vi "Dqmh Module.vi"(7 "Config":refnum<class "TAF Proj Config.lvclass">, 8 "error in (no error)":errorcluster, 11 "Library Ref":refnum<vi>) -> (0 "error out":errorcluster, 3 "Dqmh Module out":refnum<class "Dqmh Module.lvclass">)   [LabVIEW 2021, in "TAF Proj Document Type.lvlib" / "Project Parser.lvlib"]
uses:
  <vilib>/Wovalab/AntiDoc/Document Type/Add-ons/LabVIEW TAF Project/Project Parser/Project Parser.lvlib
  <vilib>/Wovalab/AntiDoc/Document Type/Add-ons/LabVIEW TAF Project/Dqmh Module/Dqmh Module.lvclass
  C:/Program Files (x86)/National Instruments/LabVIEW 2021/vi.lib/Wovalab/AntiDoc/Document Type/Add-ons/LabVIEW TAF Project/Lib/Lib.lvclass
  <vilib>/Wovalab/AntiDoc/Document Type/Add-ons/LabVIEW TAF Project/TAF Proj Config/TAF Proj Config.lvclass
  <vilib>/Wovalab/AntiDoc/Document Type/Add-ons/LabVIEW TAF Project/TAF Proj Config/TAF Proj Config.lvclass/TAF Proj Config.ctl
  <vilib>/Wovalab/AntiDoc/Document Type/Add-ons/LabVIEW TAF Project/Dqmh Module/Dqmh Module.lvclass/Dqmh Module.ctl
  <vilib>/Wovalab/AntiDoc/Document Type/Add-ons/LabVIEW TAF Project/TAF Proj Config/Read List Dqmh Default Events.vi
  <vilib>/Wovalab/AntiDoc/Document Type/Add-ons/LabVIEW TAF Project/Dqmh Module/Write Dqmh Module Type.vi
  <vilib>/Wovalab/AntiDoc/Document Type/Add-ons/LabVIEW TAF Project/Dqmh Module/Write Request Link.vi
  <vilib>/Wovalab/AntiDoc/Document Type/Add-ons/LabVIEW TAF Project/Dqmh Module/Write Broadcast Link.vi
  <vilib>/Wovalab/AntiDoc/Document Type/Add-ons/LabVIEW TAF Project/Dqmh Module/Write Request With Reply Links.vi
  <vilib>/Wovalab/AntiDoc/Document Type/Add-ons/LabVIEW TAF Project/Dqmh Module/Write Start Module Callers.vi
  <vilib>/Wovalab/AntiDoc/Document Type/Add-ons/LabVIEW TAF Project/Dqmh Module/Write Stop Module Callers.vi
  <vilib>/Wovalab/AntiDoc/Document Type/Add-ons/LabVIEW TAF Project/Dqmh Module/Write Registred Broadcast.vi
  <vilib>/Wovalab/AntiDoc/Document Type/Add-ons/LabVIEW TAF Project/Dqmh Module/Write Custom Errors.vi
  <vilib>/Wovalab/AntiDoc/Document Type/Add-ons/LabVIEW TAF Project/Dqmh Module/Write Used Requests.vi
  <vilib>/Wovalab/AntiDoc/Document Type/Add-ons/LabVIEW TAF Project/Dqmh Module/Write Used Requests With Reply.vi
  <vilib>/Wovalab/AntiDoc/Document Type/Add-ons/LabVIEW TAF Project/Dqmh Module/Write List Default Event.vi
  <vilib>/Wovalab/AntiDoc/Document Type/Add-ons/LabVIEW TAF Project/Dqmh Event/Dqmh Event.lvclass
  C:/Program Files (x86)/National Instruments/LabVIEW 2021/vi.lib/Wovalab/AntiDoc/Document Type/Add-ons/LabVIEW TAF Project/Vi/Vi.lvclass
  <vilib>/Wovalab/AntiDoc/Document Type/Add-ons/LabVIEW TAF Project/Lib/Lib.lvclass
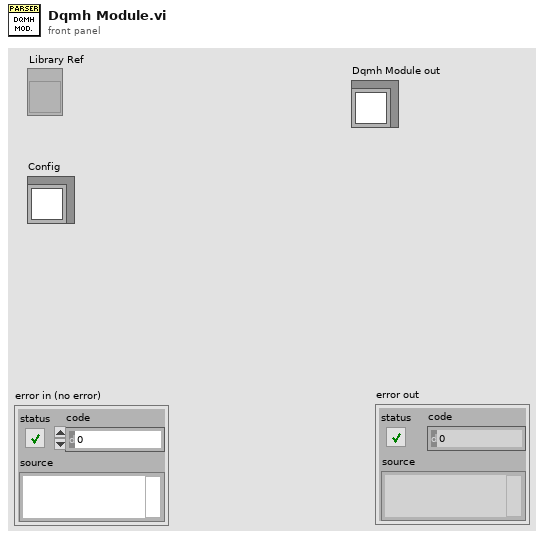
[diagram p1: front panel]
types:
  T1 = typedef "TAF Proj Document Type.lvlib/Project Parser.lvlib/Dqmh Module Info--cluster.ctl" = cluster{"Name":string, "Description":string, "Path":path, "Dqmh Module Type":T2, "Event Info":T3[], "Start Module Info":T3, "Stop Module Info":T3, "Registred Broadcast":T7[], "Custom Errors":T8[], "Used Requests":T9[], "Used Requests With Reply":T9[]}
  T2 = typedef "TAF Proj Document Type.lvlib/Project Parser.lvlib/Dqmh Module Type--enum.ctl" = enum16{"Singleton", "Cloneable"}
  T3 = typedef "TAF Proj Document Type.lvlib/Project Parser.lvlib/Dqmh Event Info--cluster.ctl" = cluster{"Vi Path":path, "Name":string, "Description":string, "Event Type":T4, "Callers":T5[], "Conpane Image":T6}
  T4 = typedef "TAF Proj Document Type.lvlib/Project Parser.lvlib/Dqmh Event Type--enum.ctl" = enum16{"Not a DQMH Event", "Request", "Request And Wait For Reply", "Broadcast"}
  T5 = typedef "TAF Proj Document Type.lvlib/Project Parser.lvlib/Dqmh Event Links--cluster.ctl" = cluster{"Owning Library":string, "Caller":string}
  T6 = typedef "imagedata.ctl" = cluster{"image type":i32, "image depth":i32, "image":u8[], "mask":u8[], "colors":u32[], "Rectangle":cluster{"left":i16, "top":i16, "right":i16, "bottom":i16}}
  T7 = typedef "TAF Proj Document Type.lvlib/Project Parser.lvlib/Module Fonctions--cluster.ctl" = cluster{"Module Name":string, "Functions":string[]}
  T8 = typedef "TAF Proj Document Type.lvlib/Project Parser.lvlib/Custom Error Info.ctl" = cluster{"Code":i32, "Name":string, "Description":string, "Owned by":string}
  T9 = typedef "TAF Proj Document Type.lvlib/Dqmh Module.lvclass/Requests Used By Module--cluster.ctl" = cluster{"Module Name":string, "Request Names":string[]}
  T10 = typedef "TAF Proj Document Type.lvlib/Project Parser.lvlib/Dqmh Event Callers--cluster.ctl" = cluster{"Event Name":string, "Caller Names":string[]}
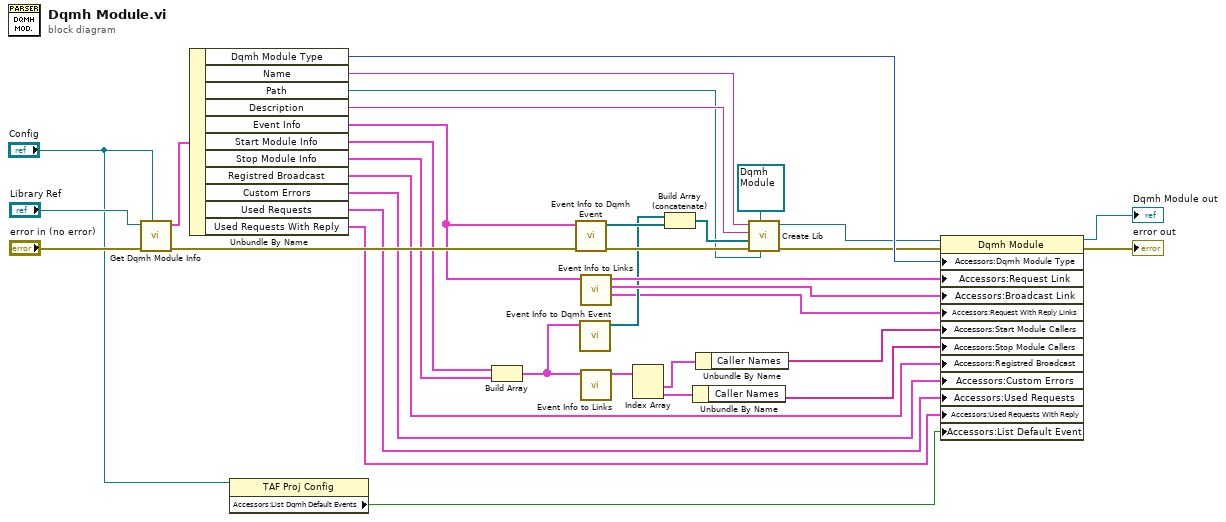
[diagram p0: block diagram]
diagram:
  n1 = call <vilib>:"Get Dqmh Module Info.vi"("Config"="Config", "error in"="error in (no error)", "Library Ref"="Library Ref") -> ("error out"=w28:errorcluster, "Dqmh Module Info"=w35:T1)  [unwired: 7 in]
  n2 = Unbundle By Name(w35) -> ("Dqmh Module Type"=w29:T2, "Name"=w33:string, "Path"=w8:path, "Description"=w32:string, "Event Info"=w26:T3[], "Start Module Info"=w21:T3, "Stop Module Info"=w20:T3, "Registred Broadcast"=w9:T7[], "Custom Errors"=w7:T8[], "Used Requests"=w2:T9[], "Used Requests With Reply"=w1:T9[])
  n3 = property class="TAF Proj Config"(reference="Config") -> ("Accessors:List Dqmh Default Events"=w3:bool)  [unwired: 1 in, 2 out]
  n4 = Build Array(w21, w20) -> (w14:T3[])
  n5 = call <vilib>:"Event Info to Dqmh Event.vi"("error in"=w28, "Event Info"=w26) -> ("error out"=w27:errorcluster, "Dqmh Event"=w13:refnum<class "Dqmh Event.lvclass">[])  [unwired: 8 in]
  n6 = call <vilib>:"Event Info to Dqmh Event.vi"("Event Info"=w14) -> ("Dqmh Event"=w11:refnum<class "Dqmh Event.lvclass">[])  [unwired: 9 in, 1 out]
  n7 = call <vilib>:"Event Info to Links.vi"("Event Info"=w26) -> ("Request With Reply Links"=w4:T10[], "Broadcast Links"=w22:T10[], "Request Links"=w23:T10[])  [unwired: 8 in]
  n8 = call <vilib>:"Event Info to Links.vi"("Event Info"=w14) -> ("Request Links"=w19:T10[])  [unwired: 8 in, 2 out]
  n9 = Index Array(array=w19) -> (element #1=w18:T10, element #2=w17:T10)  [unwired: 2 in]
  n10 = Build Array (concatenate)(w11, w13) -> (w12:refnum<class "Dqmh Event.lvclass">[])
  n11 = Unbundle By Name(w17) -> ("Caller Names"=w15:string[])
  n12 = Unbundle By Name(w18) -> ("Caller Names"=w16:string[])
  n13 = call <vilib>:"Create Lib.vi"("Path"=w8, "Lib Type"=refnum<class "Dqmh Module.lvclass"> refnum ("Dqmh Module in"), "error in"=w27, "Vis"=w12, "Description"=w32, "Name"=w33) -> ("error out"=w24:errorcluster, "Lib out"=w25:refnum<class "Dqmh Module.lvclass">)  [unwired: 4 in]
  n14 = property class="Dqmh Module"(reference=w25, error in=w24, "Accessors:Dqmh Module Type"=w29, "Accessors:Request Link"=w23, "Accessors:Broadcast Link"=w22, "Accessors:Request With Reply Links"=w4, "Accessors:Start Module Callers"=w16, "Accessors:Stop Module Callers"=w15, "Accessors:Registred Broadcast"=w9, "Accessors:Custom Errors"=w7, "Accessors:Used Requests"=w2, "Accessors:Used Requests With Reply"=w1, "Accessors:List Default Event"=w3) -> (reference out=→"Dqmh Module out":refnum<class "Dqmh Module.lvclass">, error out=→"error out":errorcluster)
